vi "Write (1D Bool).vi"(7 "count (-1: all)":i64=-1 format="%d elements", 8 "error in (no error)":errorcluster, 9 "offset (0)":u64 format="%d bytes", 10 "buffer in":bool[](array[boolean]), 11 "Pointer in":refnum<class "Pointer.lvclass">) -> (0 "error out":errorcluster, 1 "offset out":u64 format="%d bytes", 2 "buffer out":bool[](array[boolean]), 3 "Pointer out":refnum<class "Pointer.lvclass">)   [LabVIEW 2016, in "Memory Manager.lvlib" / "Pointer.lvclass"]
doc: "Writes <b>count</b> elements from the provided <b>buffer</b> to the address specified by <b>pointer + offset</b>.\n\n<b>Note:</b> This VI is <b>safe</b>.\n\nSafe means that this function evaluates the size parameter of <b>pointer</b> to ensure that is inbounds of allocated memory before peforming a memory read/write. Reading/writing more data to a pointer than it has allocated can corrupt or crash LabVIEW."
uses:
  Pointer.lvclass
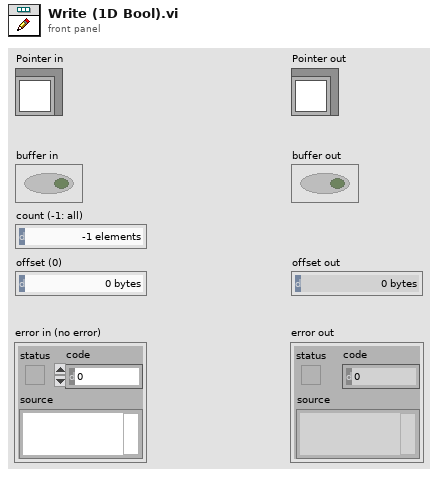
[diagram p1: front panel]
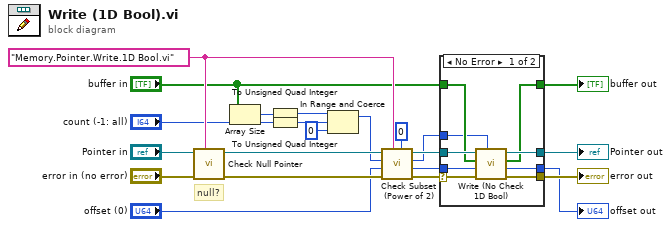
[diagram p0: block diagram]
diagram:
  w22 = "Memory.Pointer.Write.1D Bool.vi" ("source vi name")
  # "null?"
  n1 = call "Check Null Pointer.vi"("source vi name"=w22, "error in (no error)"="error in (no error)", "Pointer in"="Pointer in") -> ("error out"=w5:errorcluster, "Pointer out"=w6:refnum<class "Pointer.lvclass">)  [unwired: 7 in]
  n2 = Array Size(array="buffer in") -> (size(s)=w16:i32)
  n3 = To Unsigned Quad Integer(1:w16) -> (0:w13:u64)
  n4 = To Unsigned Quad Integer(1:"count (-1: all)") -> (0:w14:u64)
  n5 = In Range and Coerce(upper limit=w13, x=w14, lower limit=u64 0) -> (coerced(x)=w4:u64)  [unwired: 1 out]
  n6 = call "Check Subset (Power of 2).vi"("power of 2"=i16 0, "source vi name"=w22, "error in (no error)"=w5, "offset (0)"="offset (0)", "count"=w4, "Pointer in"=w6) -> ("error out"=w8:errorcluster, "offset out"=w7:u64, "count"=w3:u64, "Pointer out"=w9:refnum<class "Pointer.lvclass">)  [unwired: 2 in]
  n7 = case shown="No Error" w8 {
    selector: w8 -> [w31 w35]
    tunnel: w9 -> [w30 w34]
    tunnel: "buffer in" -> [w27 w33]
    tunnel: [w29 w35] -> w21
    tunnel: [w28 w34] -> w20
    tunnel: [w26 w33] -> w19
    tunnel: w7 -> [w25 w32]
    tunnel: [w24 w32] -> w1
    tunnel: w3 -> [w23 _]
    frame No Error {
      n8 = call "Write (No Check 1D Bool).vi"("count"=w23, "error in (no error)"=w31, "offset (0)"=w25, "buffer in"=w27, "Pointer in"=w30) -> ("error out"=w29:errorcluster, "offset out"=w24:u64, "buffer out"=w26:bool[], "Pointer out"=w28:refnum<class "Pointer.lvclass">)  [unwired: 3 in]
    }
    frame Error {
    }
  }
  "error out" <- w21
  "Pointer out" <- w20
  "buffer out" <- w19
  "offset out" <- w1
